vi "DWE Search 2D Array (String).vi"(10 "Element":string, 11 "Array":string[][](array[string])) -> (2 "element":string, 3 "Locations":i32[][](array[numeric]))   [LabVIEW 2023]
doc: "Search 2D array for a specified element (string)."
uses:
  DWE Search 2D Array (Bool).vi
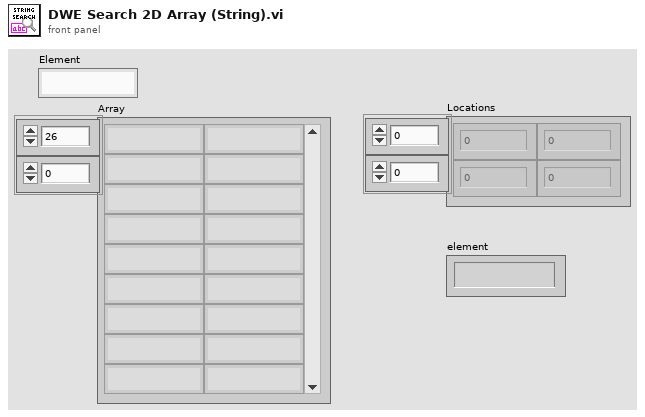
[diagram p1: front panel]
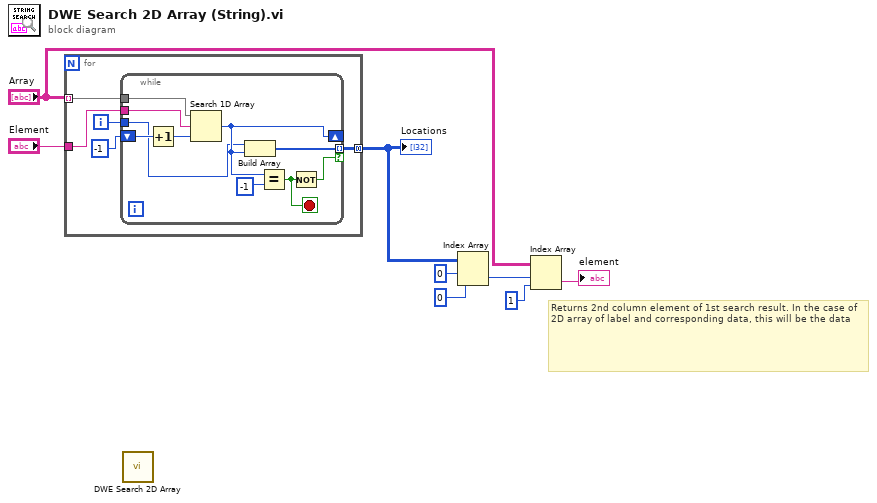
[diagram p0: block diagram]
diagram:
  # "Returns 2nd column element of 1st search result. In the case of 2D array of label and corresponding data, this will be the data"
  n1 = for {
    tunnel: "Array" -> [w13] mode=indexing
    tunnel: "Element" -> [w12]
    tunnel: [w10] -> w2 mode=concatenating
    i -> [w11]
    n2 = while {
      tunnel: w13 -> [w23]
      tunnel: w12 -> [w22]
      shift-right: [w19] -> _
      shift-left: -1 ("index of element") -> [w21]
      tunnel: w11 -> [w18]
      tunnel: [w17] -> w10 mode=indexing if=w14
      stop <- w15 stop-if-true
      n3 = Increment(x=w21) -> (x+1=w16:i32)
      n4 = Search 1D Array(1D array=w23, element=w22, start index (0)=w16) -> (index of element=w19:i32)
      n5 = Build Array(w18, w19) -> (w17:i32[])
      n6 = Equal?(x=w19, y=-1) -> (x = y?=w15:bool)
      n7 = Not(x=w15) -> (.not. x?=w14:bool)
    }
  }
  "Locations" <- w2
  n8 = call-poly "DWE Search 2D Array.vi"() -> ()  [unwired: 11 in, 1 out]
  n9 = Index Array(array=w2, index (row)=0, index (col)=0 ("disabled index (col)")) -> (element=w5:i32)
  n10 = Index Array(array="Array", index (row)=w5, index (col)=1 ("disabled index (col)")) -> (element=→"element":string)
